vi "Configure Receiver Leveling Sweep.vi"(0 "VISA resource name":refnum<visa-resource-name>, 1 "Channel (1)":i32=1, 2 "Port ( 1)":i32=1, 3 "Enable Fast IF Bandwidth (F: Disabled)":bool, 4 "IF Bandwidth (70000)":dbl=70000.0, 5 "error in (no error)":errorcluster, 6 "Enable Receiver Leveling (F: Disabled)":bool, 7 "Power Level Offset (0)":dbl, 8 "Maximum Iterations to Tolerance (5)":dbl=5.0, 9 "Tolerance Level (5)":dbl=5.0, 10 "Reference Receiver (0: R1)":i32(ring) items=["R1", "R2", "A", "B"]) -> (14 "VISA resource name out":refnum<visa-resource-name>, 19 "error out":errorcluster)   [LabVIEW 2022 SP3, in "Agilent ENA Series.lvlib"]
doc: "Configures numerous settings related to the receiver leveling sweep. \n\nNote:\nValid for E5072A only."
uses:
  Agilent ENA Series.lvlib
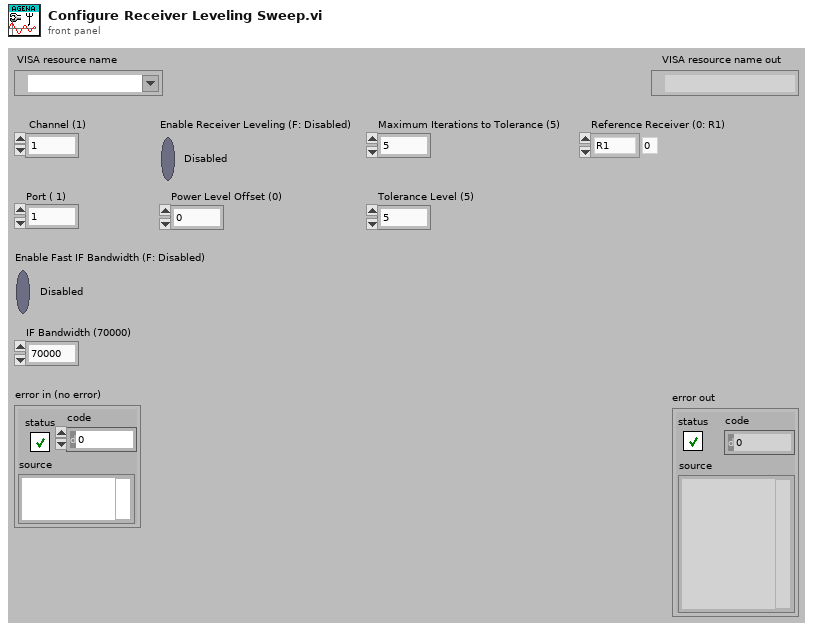
[diagram p1: front panel]
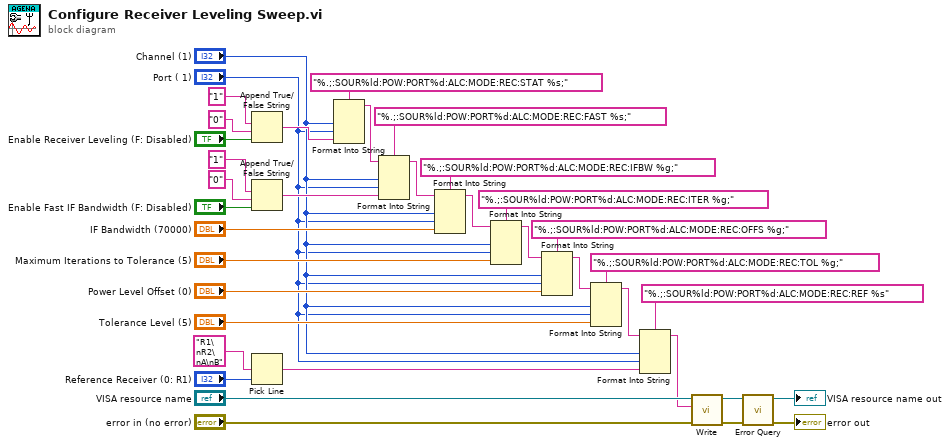
[diagram p0: block diagram]
diagram:
  n1 = Append True/False String(1:"Enable Receiver Leveling (F: Disabled)", 2:"0" ("false string"), 3:"1" ("true string")) -> (0:w29:string)  [unwired: 1 in]
  n2 = Append True/False String(1:"Enable Fast IF Bandwidth (F: Disabled)", 2:"0" ("false string"), 3:"1" ("true string")) -> (0:w25:string)  [unwired: 1 in]
  n3 = Pick Line(multi-line string="R1\nR2\nA\nB", line index="Reference Receiver (0: R1)") -> (output string=w9:string)  [unwired: 1 in]
  n4 = Format Into String(format string="%.;:SOUR%ld:POW:PORT%d:ALC:MODE:REC:STAT %s;", "Channel (1)", "Port ( 1)", w29) -> (resulting string=w24:string)  [unwired: 2 in, 1 out]
  n5 = Format Into String(format string="%.;:SOUR%ld:POW:PORT%d:ALC:MODE:REC:FAST %s;", initial string=w24, "Channel (1)", "Port ( 1)", w25) -> (resulting string=w21:string)  [unwired: 1 in, 1 out]
  n6 = Format Into String(format string="%.;:SOUR%ld:POW:PORT%d:ALC:MODE:REC:IFBW %g;", initial string=w21, "Channel (1)", "Port ( 1)", "IF Bandwidth (70000)") -> (resulting string=w6:string)  [unwired: 1 in, 1 out]
  n7 = Format Into String(format string="%.;:SOUR%ld:POW:PORT%d:ALC:MODE:REC:ITER %g;", initial string=w6, "Channel (1)", "Port ( 1)", "Maximum Iterations to Tolerance (5)") -> (resulting string=w5:string)  [unwired: 1 in, 1 out]
  n8 = Format Into String(format string="%.;:SOUR%ld:POW:PORT%d:ALC:MODE:REC:OFFS %g;", initial string=w5, "Channel (1)", "Port ( 1)", "Power Level Offset (0)") -> (resulting string=w4:string)  [unwired: 1 in, 1 out]
  n9 = Format Into String(format string="%.;:SOUR%ld:POW:PORT%d:ALC:MODE:REC:TOL %g;", initial string=w4, "Channel (1)", "Port ( 1)", "Tolerance Level (5)") -> (resulting string=w13:string)  [unwired: 1 in, 1 out]
  n10 = Format Into String(format string="%.;:SOUR%ld:POW:PORT%d:ALC:MODE:REC:REF %s", initial string=w13, "Channel (1)", "Port ( 1)", w9) -> (resulting string=w3:string)  [unwired: 1 in, 1 out]
  n11 = call "Write.vi"("error in (no error)"="error in (no error)", "String ()"=w3, "VISA resource name"="VISA resource name") -> ("error out"=w2:errorcluster, "VISA resource name out"=w35:refnum<visa-resource-name>)  [unwired: 6 in, 1 out]
  n12 = call "Error Query.vi"("error in (no error)"=w2, "VISA resource name"=w35) -> ("error out"=→"error out":errorcluster, "VISA resource name out"=→"VISA resource name out":refnum<visa-resource-name>)  [unwired: 6 in, 2 out]
